vi "PIO Read Benchmark.vi"() -> ()   [LabVIEW 2016]
uses:
  Source/GE 5565PIORC/GE 5565PIORC.lvclass
  <vilib>/platform/TimedLoop/XDataNode/XDataNode.xnode
  <vilib>/Platform/TimedLoop/XDataNode/nitl_modes.ctl
  <vilib>/Platform/TimedLoop/XDataNode/XDNodeRunTimeDep.lvlib
  <vilib>/Platform/TimedLoop/XDataNode/wakeup.ctl
  <vilib>/Platform/TimedLoop/XDataNode/timing_clust.ctl
  Source/GE 5565PIORC/VIs/PIO/Polymorphic VIs/PIO.Read (U8).vi
panel:
  in  "count":u32
  out "Duration":dbl
  in  "VISA resource name":refnum<visa-resource-name>
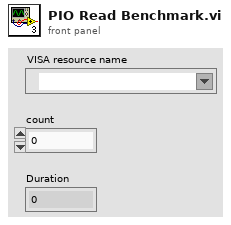
[diagram p1: front panel]
types:
  T1 = typedef "XDNodeRunTimeDep.lvlib/timing_clust.ctl" = cluster{"Expected End [f-1]":u64, "Actual End [f-1]":u64, "Finished Late? [f-1]":bool, "Expected End [i-1]":u64, "Actual End [i-1]":u64, "Finished Late? [i-1]":bool, "Expected Start [i]":u64, "Actual Start [i]":u64, "Expected Start [f]":u64, "Actual Start [f]":u64, "Source Name":string, "Structure Name":string, "Period":i64, "Deadline":i64, "Offset":i64, "Start":i64, "Priority":i32, "Timeout":i32, "Mode":T2, "Wakeup Reason":T3, "Error":errorcluster, "Source Type":string, "Secondary Source Type":string, "Global End Time":u64, "Global Start Time":u64, "Frame Duration":u64, "Iteration Duration":u64, "Assigned CPU":i32, "I/O Scan Engine Mode":u32}
  T2 = typedef "XDNodeRunTimeDep.lvlib/nitl_modes.ctl" = enum32{"No Change", "Process missed periods, maintain original phase", "Discard missed periods, maintain original phase", "Process missed periods, ignore original phase", "Discard missed periods, ignore original phase"}
  T3 = typedef "XDNodeRunTimeDep.lvlib/wakeup.ctl" = enum32{"Normal", "Aborted", "Asynchronous wakeup", "Timing source error", "Timed loop error", "Timeout"}
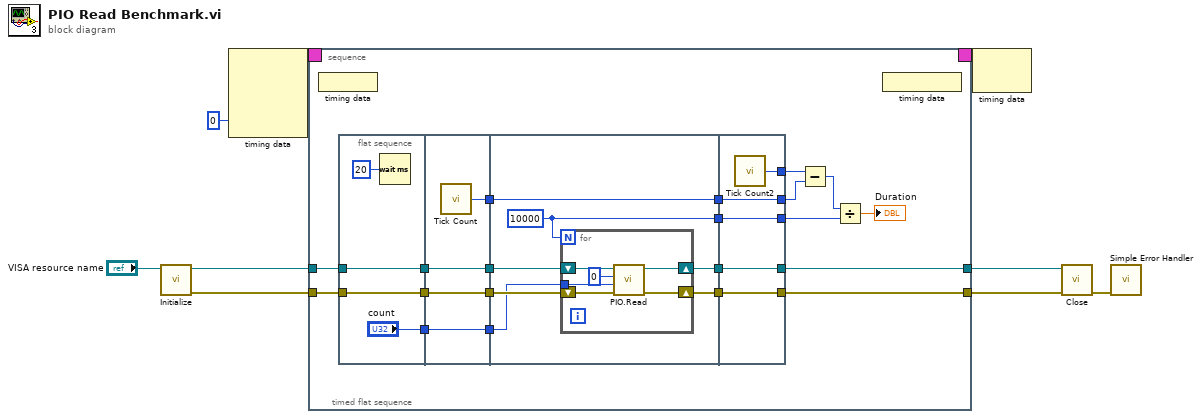
[diagram p0: block diagram]
diagram:
  n1 = call "Initialize.vi"("VISA resource name"="VISA resource name") -> ("error out"=w3:errorcluster, "GE 5565PIORC"=w4:refnum<class "GE 5565PIORC.lvclass">)  [unwired: 9 in]
  n2 = node-c288(0 ("Processor")) -> (w7:T1)  [unwired: 3 in]
  n3 = timed-sequence {
    timing: w7 -> [_]
    timing-out: [_] -> w6
    tunnel: w4 -> [w13]
    tunnel: w3 -> [w12]
    tunnel: [w11] -> w2
    tunnel: [w10] -> w1
    n4 = timed-flat-sequence {
      tunnel: w13 -> [w29]
      tunnel: w12 -> [w28]
      tunnel: [w17] -> w11
      tunnel: [w16] -> w10
      n5 = node-c288() -> ()  [unwired: 1 in]
      n6 = flat-sequence {
        tunnel: w29 -> [w36]
        tunnel: w28 -> [w35]
        tunnel: [w36] -> w26
        tunnel: [w35] -> w24
        tunnel: ["count"] -> w15
        tunnel: [w41] -> w33
        tunnel: [w40] -> w27
        tunnel: w26 -> [w40]
        tunnel: [w39] -> w25
        tunnel: w24 -> [w39]
        tunnel: w15 -> [w38]
        tunnel: [w38] -> w14
        tunnel: w33 -> [w48]
        tunnel: [w48] -> w32
        tunnel: w27 -> [w47]
        tunnel: w25 -> [w46]
        tunnel: [w45] -> w23
        tunnel: [w44] -> w22
        tunnel: [w43] -> w21
        tunnel: w14 -> [w42]
        tunnel: [w59] -> w31
        tunnel: [w58] -> w30
        tunnel: w32 -> [w58]
        tunnel: w23 -> [w57]
        tunnel: w22 -> [w56]
        tunnel: [w57] -> w17
        tunnel: [w56] -> w16
        tunnel: w21 -> [w55]
        tunnel: [w55] -> w19
        frame #0 {
          n7 = Wait (ms)(milliseconds to wait=u32 20) -> ()  [unwired: 1 out]
        }
        frame #1 {
          n8 = call "Tick Count"() -> ("Tick Count(uSec)"=w41:u32)
        }
        frame #2 {
          w43 = 10000
          n9 = for {
            N: w43 -> [_]
            shift-right: [w53] -> w45
            shift-left: w47 -> [w54]
            shift-right: [w51] -> w44
            shift-left: w46 -> [w52]
            tunnel: w42 -> [w50]
            n10 = call-poly "PIO.Read.vi"("error in (no error)"=w52, 9:w50, "offset"=u32 0, "GE 5565PIORC in"=w54) -> ("error out"=w51:errorcluster, "GE 5565PIORC out"=w53:refnum<class "GE 5565PIORC.lvclass">)  [unwired: 5 in, 1 out]
          }
        }
        frame #3 {
          n11 = call "Tick Count2"() -> ("Tick Count(uSec)"=w59:u32)
        }
      }
      n12 = Subtract(x=w31, y=w30) -> (x-y=w20:u32)
      n13 = Divide(x=w20, y=w19) -> (x/y=→"Duration":dbl)
      n14 = node-c288() -> ()  [unwired: 1 out]
    }
  }
  n15 = node-c288(w6) -> ()  [unwired: 1 out]
  n16 = call "Close.vi"("error in (no error)"=w1, "GE 5565PIORC in"=w2) -> ("error out"=w8:errorcluster)  [unwired: 8 in, 1 out]
  n17 = call <vilib>:"Simple Error Handler.vi"("error in (no error)"=w8) -> ()  [unwired: 4 in, 5 out]
